vi "processResult.vi"(8 "error in":errorcluster, 10 "TestResult in":refnum<class "TestResult.lvclass">, 11 "TextTestRunner in":refnum<class "TextTestRunner.lvclass">) -> (0 "error out":errorcluster, 2 "TestResult out":refnum<class "TestResult.lvclass">, 3 "TextTestRunner out":refnum<class "TextTestRunner.lvclass">)   [LabVIEW 2011, in "TextTestRunner.lvclass"]
uses:
  TextTestRunner.lvclass
  TestResult/TestResult.lvclass
  _TextTestResult/_TextTestResult.lvclass
  TestRunner/TestRunner.lvclass
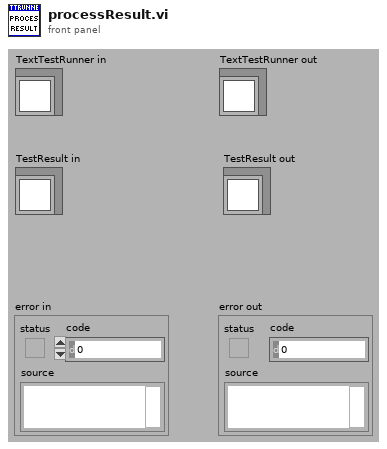
[diagram p1: front panel]
types:
  T1 = typedef "TestResult.lvclass/failure.ctl" = cluster{"test":refnum<class>, "error":errorcluster}
  T2 = typedef "TestResult.lvclass/errors.ctl" = T3[]
  T3 = typedef "TestResult.lvclass/error.ctl" = cluster{"test":refnum<class>, "error":errorcluster}
  T4 = typedef "TestResult.lvclass/skipped.ctl" = T5[]
  T5 = typedef "TestResult.lvclass/skip.ctl" = cluster{"test":refnum<class>, "error":errorcluster}
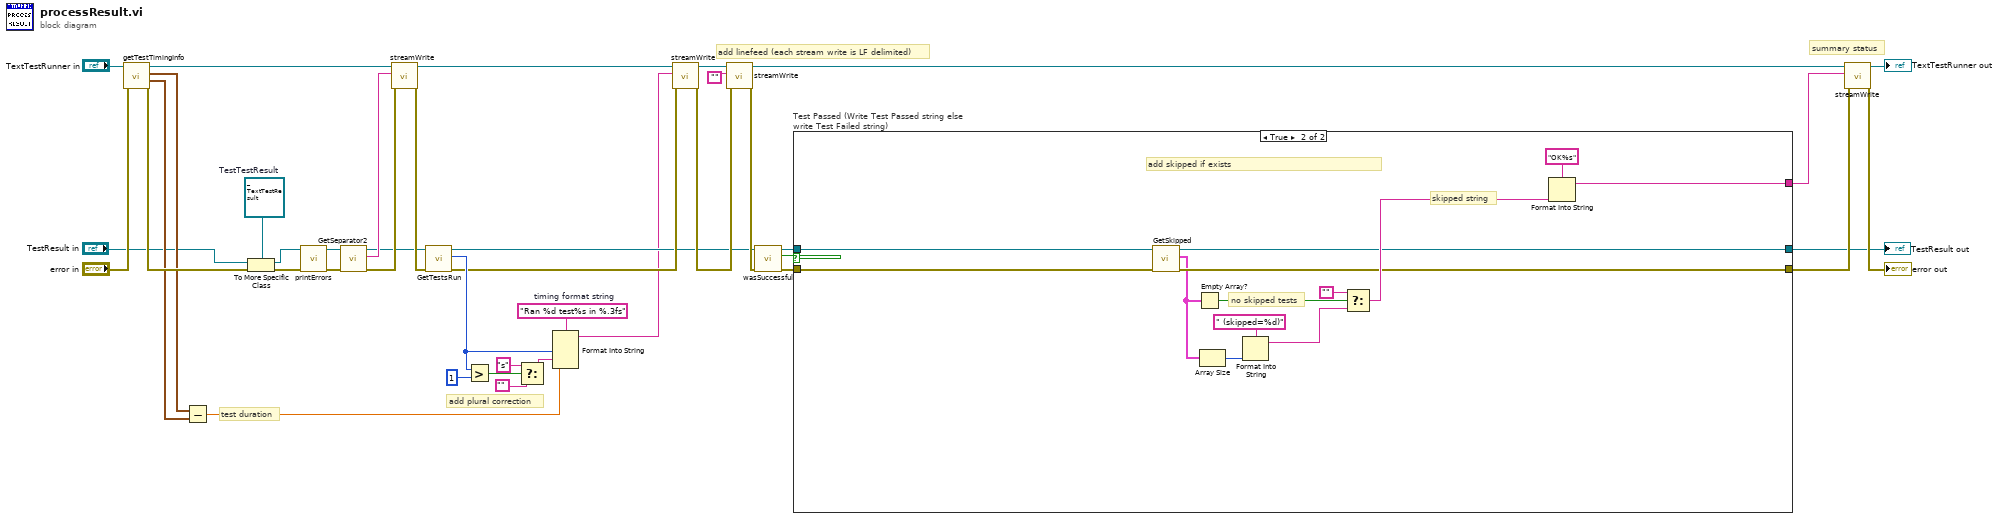
[diagram p0: block diagram]
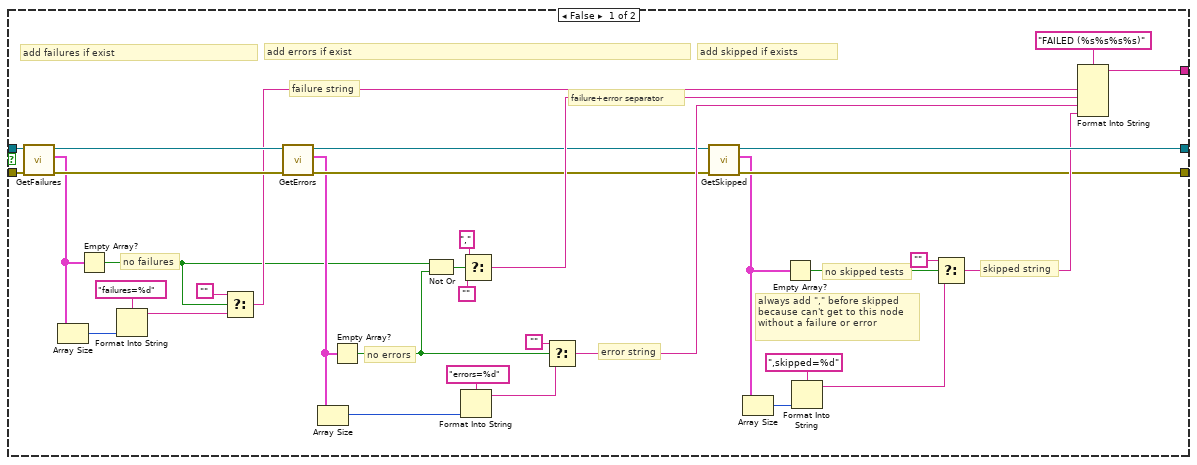
[diagram p2: hidden frame]
diagram:
  w15 = refnum<class "_TextTestResult.lvclass"> refnum  # TestTestResult
  w41 = "Ran %d test%s in %.3fs"  # timing format string
  # "add plural correction"
  # "summary status"
  # "add linefeed (each stream write is LF delimited)"
  # "test duration"
  n1 = call "getTestTimingInfo.vi"("error in"="error in", "TestRunner in"="TextTestRunner in") -> ("error out"=w6:errorcluster, "Start Time"=w4:timestamp, "Stop Time"=w5:timestamp, "TestRunner out"=w8:refnum<class "TextTestRunner.lvclass">)  [unwired: 6 in]
  n2 = Subtract(x=w5, y=w4) -> (x-y=w40:dbl)
  n3 = To More Specific Class(target class=w15, reference="TestResult in", error in=w6) -> (specific class reference=w1:refnum<class "_TextTestResult.lvclass">, error out=w16:errorcluster)
  n4 = call-dynamic "printErrors.vi"("error in (no error)"=w16, "TestTestResult in"=w1) -> ("error out"=w18:errorcluster, "TestTestResult out"=w17:refnum<class "_TextTestResult.lvclass">)  [unwired: 8 in]
  n5 = call-dynamic "GetSeparator2.vi"("error in (no error)"=w18, "TestTestResult in"=w17) -> ("error out"=w29:errorcluster, "separator2"=w30:string, "TestTestResult out"=w27:refnum<class "_TextTestResult.lvclass">)  [unwired: 7 in]
  n6 = call-dynamic "streamWrite.vi"("error in (no error)"=w29, "String"=w30, "TextTestRunner in"=w8) -> ("error out"=w28:errorcluster, "TextTestRunner out"=w20:refnum<class "TextTestRunner.lvclass">)  [unwired: 7 in]
  n7 = call-dynamic "GetTestsRun.vi"("error in (no error)"=w28, "TestResult in"=w27) -> ("error out"=w25:errorcluster, "testsRun"=w39:u32, "TestResult out"=w22:refnum<class "_TextTestResult.lvclass">)  [unwired: 7 in]
  n8 = Greater?(x=w39, y=u32 1) -> (0:w37:bool)
  n9 = Select(t="s", s=w37, f="") -> (s? t:f=w34:string)
  n10 = Format Into String(format string=w41, w39, w34, w40) -> (resulting string=w21:string)  [unwired: 2 in, 1 out]
  n11 = call-dynamic "streamWrite.vi"("error in (no error)"=w25, "String"=w21, "TextTestRunner in"=w20) -> ("error out"=w24:errorcluster, "TextTestRunner out"=w19:refnum<class "TextTestRunner.lvclass">)  [unwired: 7 in]
  n12 = call-dynamic "streamWrite.vi"("error in (no error)"=w24, "String"="", "TextTestRunner in"=w19) -> ("error out"=w23:errorcluster, "TextTestRunner out"=w14:refnum<class "TextTestRunner.lvclass">)  [unwired: 7 in]
  n13 = call-dynamic "wasSuccessful.vi"("error in (no error)"=w23, "TestResult in"=w22) -> ("error out"=w31:errorcluster, "successful?"=w33:bool, "TestResult in"=w32:refnum<class "_TextTestResult.lvclass">)  [unwired: 7 in]
  n14 = case "Test Passed (Write Test Passed string else write Test Failed string)" shown="True" w33 {
    tunnel: w32 -> [w66 w84]
    tunnel: w31 -> [w65 w85]
    tunnel: [w61 w83] -> w3
    tunnel: [w57 w82] -> w11
    tunnel: [w58 w81] -> w10
    frame False {
      # "no skipped tests"
      # "skipped string"
      # "always add \",\" before skipped because can't get to this node without a failure or error"
      # "failure+error separator"
      # "error string"
      # "failure string"
      # "no errors"
      # "no failures"
      # "add errors if exist"
      # "add failures if exist"
      # "add skipped if exists"
      n15 = call-dynamic "GetFailures.vi"("error in (no error)"=w65, "TestResult in"=w66) -> ("error out"=w71:errorcluster, "failures"=w56:T1[], "TestResult out"=w72:refnum<class "_TextTestResult.lvclass">)  [unwired: 7 in]
      n16 = Array Size(array=w56) -> (size(s)=w75:i32)
      n17 = Empty Array?(array=w56) -> (empty?=w50:bool)
      n18 = Format Into String(format string="failures=%d" ("String"), w75) -> (resulting string=w54:string)  [unwired: 2 in, 1 out]
      n19 = Select(t="", s=w50, f=w54) -> (s? t:f=w69:string)
      n20 = call-dynamic "GetErrors.vi"("error in (no error)"=w71, "TestResult in"=w72) -> ("error out"=w63:errorcluster, "Errors"=w53:T2, "TestResult out"=w62:refnum<class "_TextTestResult.lvclass">)  [unwired: 7 in]
      n21 = Array Size(array=w53) -> (size(s)=w73:i32)
      n22 = Empty Array?(array=w53) -> (empty?=w49:bool)
      n23 = Not Or(1:w49, 2:w50) -> (0:w48:bool)
      n24 = Format Into String(format string="errors=%d" ("String"), w73) -> (resulting string=w51:string)  [unwired: 2 in, 1 out]
      n25 = Select(t=",", s=w48, f="") -> (s? t:f=w68:string)
      n26 = Select(t="", s=w49, f=w51) -> (s? t:f=w67:string)
      n27 = call-dynamic "GetSkipped.vi"("error in (no error)"=w63, "TestResult in"=w62) -> ("error out"=w57:errorcluster, "Skipped"=w45:T4, "TestResult in"=w61:refnum<class "_TextTestResult.lvclass">)  [unwired: 7 in]
      n28 = Array Size(array=w45) -> (size(s)=w64:i32)
      n29 = Empty Array?(array=w45) -> (empty?=w44:bool)
      n30 = Format Into String(format string=",skipped=%d" ("String"), w64) -> (resulting string=w42:string)  [unwired: 2 in, 1 out]
      n31 = Select(t="", s=w44, f=w42) -> (s? t:f=w59:string)
      n32 = Format Into String(format string="FAILED (%s%s%s%s)" ("String"), w69, w68, w67, w59) -> (resulting string=w58:string)  [unwired: 2 in, 1 out]
    }
    frame True {
      # "skipped string"
      # "no skipped tests"
      # "add skipped if exists"
      n33 = call-dynamic "GetSkipped.vi"("error in (no error)"=w85, "TestResult in"=w84) -> ("error out"=w82:errorcluster, "Skipped"=w80:T4, "TestResult in"=w83:refnum<class "_TextTestResult.lvclass">)  [unwired: 7 in]
      n34 = Empty Array?(array=w80) -> (empty?=w79:bool)
      n35 = Array Size(array=w80) -> (size(s)=w89:i32)
      n36 = Format Into String(format string=" (skipped=%d)" ("String"), w89) -> (resulting string=w77:string)  [unwired: 2 in, 1 out]
      n37 = Select(t="", s=w79, f=w77) -> (s? t:f=w86:string)
      n38 = Format Into String(format string="OK%s", w86) -> (resulting string=w81:string)  [unwired: 2 in, 1 out]
    }
  }
  "TestResult out" <- w3
  n39 = call-dynamic "streamWrite.vi"("error in (no error)"=w11, "String"=w10, "TextTestRunner in"=w14) -> ("error out"=→"error out":errorcluster, "TextTestRunner out"=→"TextTestRunner out":refnum<class "TextTestRunner.lvclass">)  [unwired: 7 in]
